vi "CalibrateDistanceCameraSyringe.vi"(5 ".NET Refnum in":refnum<k24>, 6 "error in":errorcluster, 7 "Image Feed":T6, 8 "Template Path":path=path "C:/Users/Aerotech/Documents/BNL_ThermomechanicalStave/1_ModulePlacement", 9 "um/pix resolution":dbl=1.5800403213058958, 10 "Axis speeds (mm/s)":T5={"vX [mm]"=20.0, "vY [mm]"=20.0, "vZ [mm] "=20.0}, 11 "Path to save collected images":path=path "C:/Users/Aerotech/cernbox/BNL/Stave Assembly Records/2017-05-12") -> (0 "X/Y difference (CAMERA - SYRINGE)":dbl[][](array[numeric])=[[-130.04319981335846, 7.799950189407227], [-133.07688928470915, 5.629009425384126]], 3 "XYZ .NET Refnum out":refnum<k24>, 4 "error out":errorcluster={"status"=FALSE, "code"=1073676418, "source"="VISA Close in CalibrateDistanceCameraSyringe.vi"})   [LabVIEW 2016]
uses:
  <vilib>/LabVIEW Interface for Arduino/Type Defs/Arduino Resource.ctl
  <vilib>/LabVIEW Interface for Arduino/Type Defs/Board Type.ctl
  C:/Users/Aerotech/Documents/BNL_ThermomechanicalStave/AerotechLibraries/Bin/Aerotech.A3200.dll
  AerotechLibraries/Bin/Aerotech.A3200.dll
  <vilib>/vision/Measure.llb/Edge Options.ctl
  <vilib>/vision/Measure.llb/Edge Polarity.ctl
  <vilib>/vision/Image Controls.llb/IMAQ Image.ctl
  <vilib>/userdefined/High Color/IMAQdx.ctl
  <vilib>/LabVIEW Interface for Arduino/Type Defs/Pin Mode.ctl
  <vilib>/LabVIEW Interface for Arduino/LabVIEW Interface for Arduino.lvlib
  <vilib>/vision/NI_Vision_Development_Module.lvlib
  <vilib>/vision/driver/NI_Vision_Acquisition_Software.lvlib
panel:
  in  "?":T1(tab)=enum."Results and Error Handling"
  in  "Off stave position":T2={"X [mm]"=250.0, "Y [mm]"=-110.0, "Z [mm] "=26.0}
  in  "Estimate distance x":dbl=132.0
  in  "Estimate distance y":dbl=4.0
  in  "Camera Z":dbl=-24.0
  out "XYZ Stage Control":refnum<k24>
  out "Arduino Resource":T3={"VISA resource"="COM4", "Board Type"=enum."Uno", "Connection Type"=enum."USB / Serial", "Bytes Per Packet (15)"=15}
  in  "Digital I/O Pin":u8=7
  in  "Lowest Z Position":dbl=46.0
  out "Template Image":T6
  out "Camera session out":T7="cam1"
  in  "Camera Name":T7="cam1" caption="IMAQdx Session"
  in  "Testing?":bool
  in  "Circle Finding Options":T10={"Search  Direction"=1, "Edge Options"={"Edge Polarity"=2, "Kernel Size"=3, "Width"=3, "Minimum Edge Strength"=10.0, "Interpolation Type"=enum."Bilinear Fixed", "Data Processing Method"=enum."Median"}, "Show Search Area"=FALSE, "Show Search Lines"=FALSE, "Show Edges Found"=FALSE, "Show Result"=TRUE, "Search Area Color"=65280, "Search Lines Color"=255, "Edge Locations Color"=16776960, "Result Color"=65511, "Overlay Group Name"=""} {"Search  Direction" items=["Outside to Inside", "Inside to Outside"]; "Edge Options"."Edge Polarity" items=["All Edges", "Rising Edges", "Falling Edges"]; "Edge Options"."Minimum Edge Strength" format="%.2f"; "Edge Options"."Width" step=2; "Edge Options"."Kernel Size" step=2}
  in  "Circle ROI Descriptor":T11={"Global Rectangle"=[675, 567, 1751, 1642], "Contours"=[{"ID"=enum."External", "Type"=7, "Coordinates"=[1212, 1104, 85, 537, 0, 0]}]} {"Contours"."Type" items=["No Selection", "Point", "Line", "Rectangle", "Oval", "Polygon", "Freehand Region", "Annulus", "Unused2", "Unused3", "Broken Line", "Freehand Line", "Rotated Rectangle"]}
  in  "Pattern Match Settings":T12={"Algorithm"=2, "Number of Matches Requested"=1, "Minimum Match Score"=100.0, "SubPixel Accuracy"=TRUE, "Rotation Angle Ranges"=[{"Start"=0.0, "End"=360.0}], "Show Search Area"=FALSE, "Show Result"=TRUE} {"Rotation Angle Ranges"."End" format="%.1f"; "Rotation Angle Ranges"."Start" format="%.1f"; "Minimum Match Score" min=0 max=1000 format="%.2f"; "Number of Matches Requested" min=1; "Algorithm" items=["All", "Low Discrepancy Sampling", "Grayscale Value Pyramid", "Gradients Pyramid"]}
  in  "Circle Fit Options":T13={"Process"=enum."Get Best Edge", "Step Size"=3.0, "Max Pixel Radius"=3}
  in  "Fit Circle?":bool
  out "Number of Matches":i32=1
  out "Estimate location":T2={"X [mm]"=118.0, "Y [mm]"=-106.0, "Z [mm] "=-24.0}
  out "pixels x":dbl=1920.0
  out "pixels y":dbl=1374.0
  out "Dot image":T6(plugin-control)
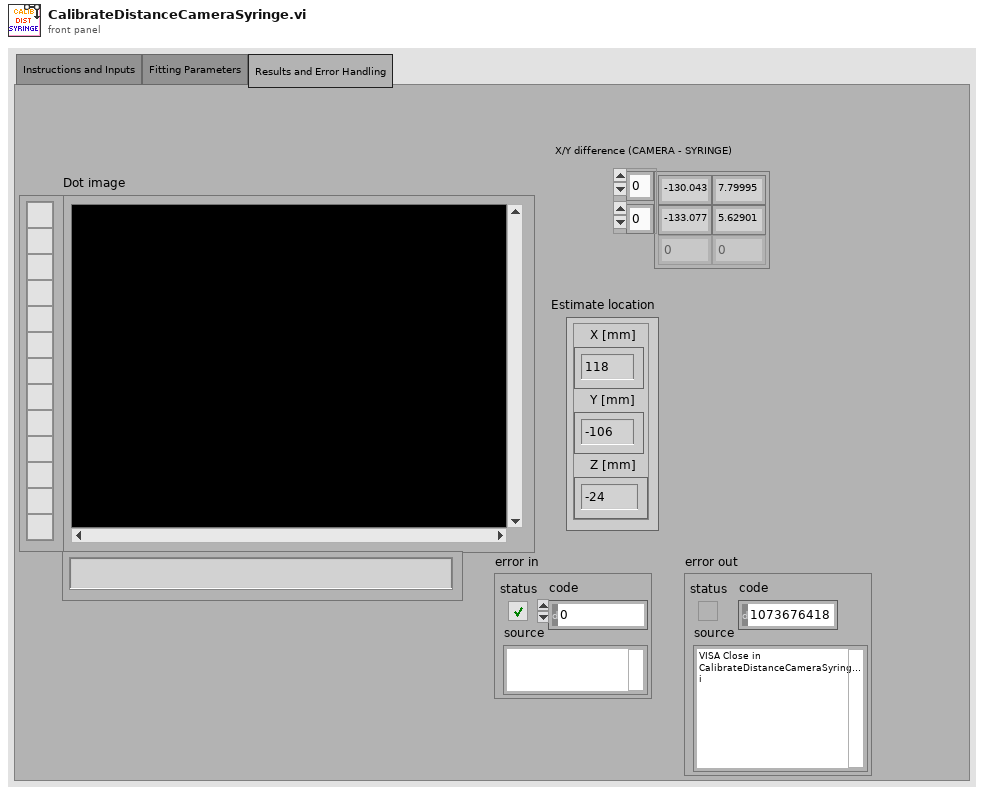
[diagram p1: front panel]
types:
  T1 = enum32{"Instructions and Inputs", "Fitting Parameters", "Results and Error Handling"}
  T2 = cluster{"X [mm]":dbl, "Y [mm]":dbl, "Z [mm] ":dbl}
  T3 = typedef "LabVIEW Interface for Arduino.lvlib/Arduino Resource.ctl" = cluster{"VISA resource":refnum<visa-resource-name>, "Board Type":T4, "Connection Type":enum8{"USB / Serial"}, "Bytes Per Packet (15)":u8}
  T4 = typedef "LabVIEW Interface for Arduino.lvlib/Board Type.ctl" = enum16{"Uno", "Dimuelanove w/Atmega 328", "Mega 2560"}
  T5 = cluster{"vX [mm]":dbl, "vY [mm]":dbl, "vZ [mm] ":dbl}
  T6 = typedef "IMAQ Image.ctl" = refnum<image>
  T7 = typedef "IMAQdx.ctl" = refnum<k21>
  T8 = typedef "Edge Options.ctl" = cluster{"Edge Polarity":T9, "Kernel Size":u32, "Width":u32, "Minimum Edge Strength":sgl, "Interpolation Type":enum32{"Zero Order", "Bilinear", "Quadratic", "Cubic", "Bilinear Fixed"}, "Data Processing Method":enum32{"Average", "Median"}}
  T9 = typedef "Edge Polarity.ctl" = u32
  T10 = cluster{"Search  Direction":u32, "Edge Options":T8, "Show Search Area":bool, "Show Search Lines":bool, "Show Edges Found":bool, "Show Result":bool, "Search Area Color":u32, "Search Lines Color":u32, "Edge Locations Color":u32, "Result Color":u32, "Overlay Group Name":string}
  T11 = cluster{"Global Rectangle":i32[], "Contours":cluster{"ID":enum32{"External", "Internal"}, "Type":u32, "Coordinates":i32[]}[]}
  T12 = cluster{"Algorithm":i32, "Number of Matches Requested":i32, "Minimum Match Score":sgl, "SubPixel Accuracy":bool, "Rotation Angle Ranges":cluster{"Start":sgl, "End":sgl}[], "Show Search Area":bool, "Show Result":bool}
  T13 = cluster{"Process":enum16{"Get First Edge", "Get First + Last Edge", "Get All Edges", "Get Best Edge"}, "Step Size":dbl, "Max Pixel Radius":i32}
  T14 = typedef "LabVIEW Interface for Arduino.lvlib/Pin Mode.ctl" = enum8{"Input", "Output"}
  T15 = typedef "Image Type" = u32
  T16 = cluster{"X [mm]":dbl, "Y [mm]":dbl, "Lowest Z Position":dbl}
  T17 = cluster{"Image Dst Out":T6, "Axis speeds (mm/s)":cluster{"vX [mm]":dbl, "vY [mm]":dbl, "vZ [mm] ":dbl}, ".NET Refnum out":refnum<k24>}
  T18 = cluster{"Captured positions":dbl[][], "XYZ .NET Refnum out":refnum<k24>}
  T19 = cluster{"Position":cluster{"x":sgl, "y":sgl}, "Angle":sgl, "Scale":sgl, "Score":sgl, "Bounding Box":cluster{"x":sgl, "y":sgl}[]}[]
  T20 = cluster{"Position":cluster{"x":sgl, "y":sgl}, "Angle":sgl, "Scale":sgl, "Score":sgl, "Bounding Box":cluster{"x":sgl, "y":sgl}[]}
  T21 = cluster{"Global Rectangle":i32[], cluster{"ID":enum32{"External", "Internal"}, "Type":u32, "Coordinates":i32[]}[]}
  T22 = cluster{"Center (Pixels)":cluster{"X":sgl, "Y":sgl}, "Radius (Pixels)":dbl, "Center (Real-World)":cluster{"X":sgl, "Y":sgl}, "Radius (Real-World)":dbl, "Roundness (Real-World)":dbl, "Average Strength":dbl, "Average SNR (dB)":dbl}
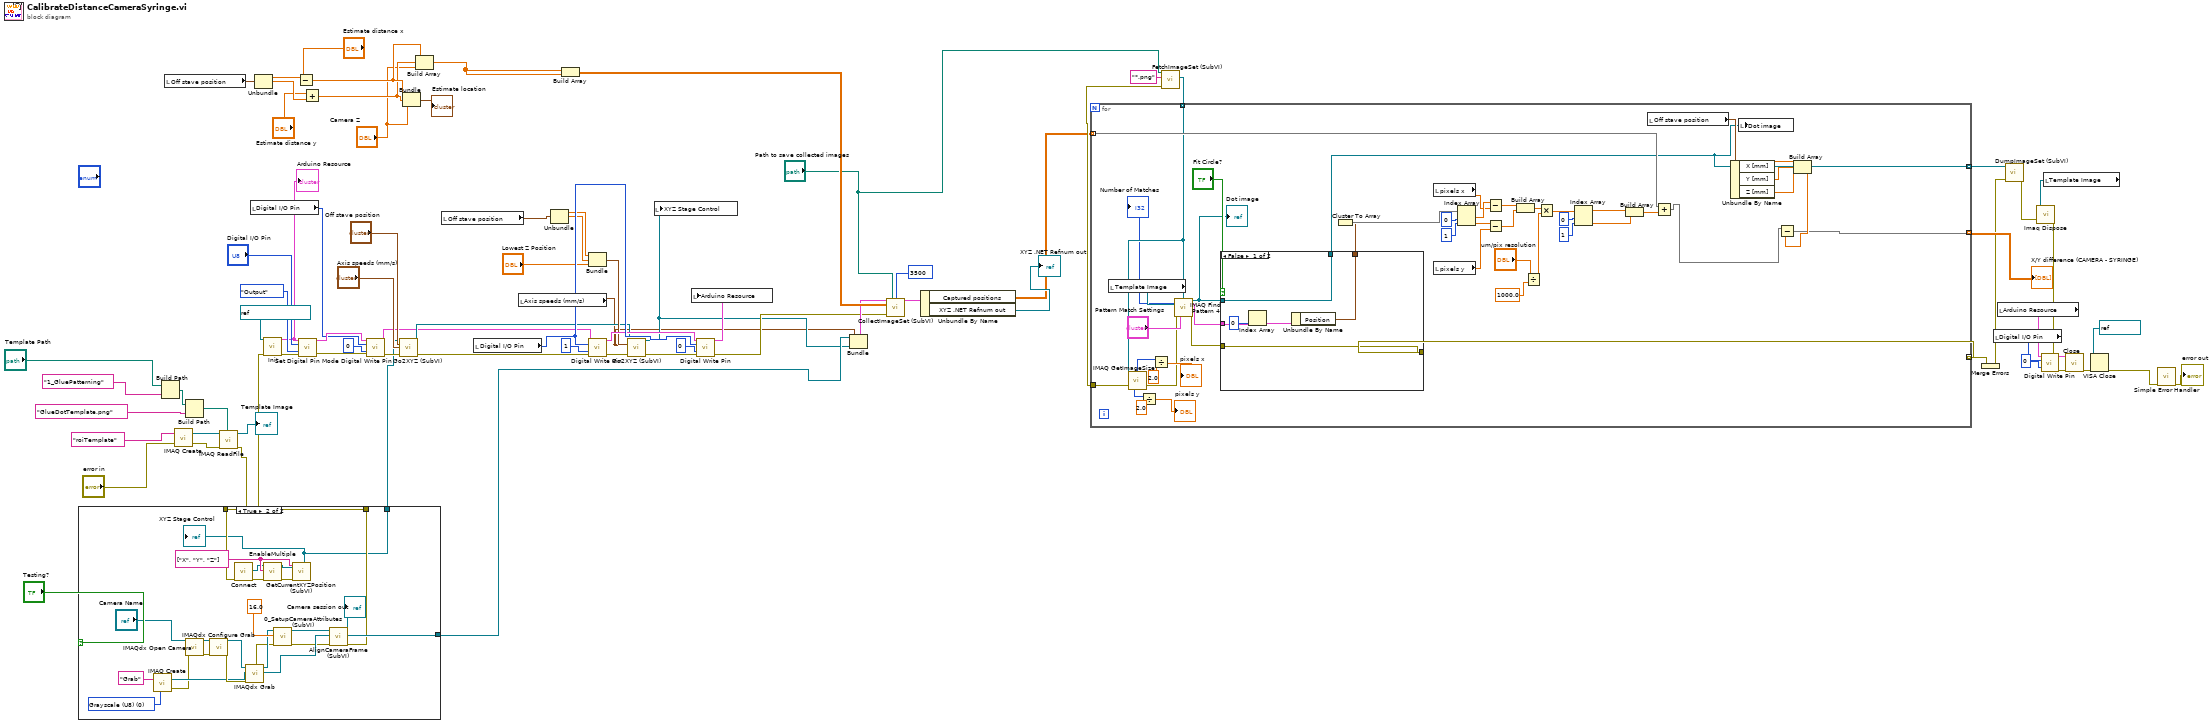
[diagram p0: block diagram]
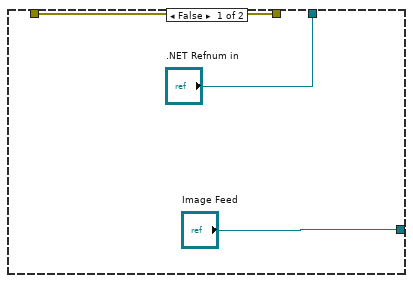
[diagram p2: hidden frame]
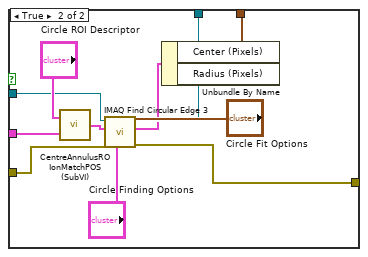
[diagram p3: hidden frame]
diagram:
  n1 = Build Path(base path="Template Path", name or relative path="1_GluePatterning") -> (appended path=w44:path)
  n2 = local read "Off stave position"() -> (w58:T2)
  n3 = call "IMAQ Create"("Image Name"="roiTemplate", "error in (no error)"="error in") -> ("New Image"=w47:T6, "error out"=w48:errorcluster)  [unwired: 3 in]
  n4 = Build Path(base path=w44, name or relative path="GlueDotTemplate.png") -> (appended path=w42:path)
  n5 = call "IMAQ ReadFile"("File Path"=w42, "error in (no error)"=w48, "Image"=w47) -> ("error out"=w22:errorcluster, "Image Out"=→"Template Image":T6)  [unwired: 4 in, 3 out]
  n6 = case shown="True" "Testing?" {
    tunnel: ["Image Feed" w97] -> w31
    tunnel: w22 -> [w84 w89]
    tunnel: [w84 w88] -> w4
    tunnel: [".NET Refnum in" w85] -> w3
    frame False {
    }
    frame True {
      w87 = T15 0 items=["Grayscale (U8)", "Grayscale (I16)", "Grayscale (SGL)", "Complex (CSG)", "RGB (U32)", "HSL (U32)", "RGB (U64)", "Grayscale (U16)"] ("Image Type")
      w93 = string[] ["X", "Y", "Z"] ("Axes Names")
      n7 = call "IMAQ Create"("Image Name"="Grab", "Image Type"=w87) -> ("New Image"=w96:T6, "error out"=w94:errorcluster)  [unwired: 3 in]
      n8 = call <vilib>:"IMAQdx Open Camera.vi"("error in"=w94, "Session In"="Camera Name") -> ("error out"=w107:errorcluster, "Session Out"=w108:T7)  [unwired: 1 in, 7 out]
      n9 = call <vilib>:"IMAQdx Configure Grab.vi"("error in"=w107, "Session In"=w108) -> ("error out"=w100:errorcluster, "Session Out"=w105:T7)  [unwired: 8 out]
      n10 = call "Connect.vi"("error in (no error)"=w89) -> ("error out"=w91:errorcluster, "controller"=w92:refnum<k24>)  [unwired: 9 in]
      n11 = call <vilib>:"IMAQdx Grab.vi"("error in"=w100, "Image In"=w96, "Session In"=w105) -> ("error out"=w99:errorcluster, "Image Out"=w102:T6, "Session Out"=w104:T7)  [unwired: 1 in, 5 out]
      n12 = call "EnableMultiple.vi"("error in (no error)"=w91, "axis names"=w93, "controller in"=w92) -> ("error out"=w90:errorcluster, "controller out"=w86:refnum<k24>)  [unwired: 7 in]
      n13 = call "0_SetupCameraAttributes (SubVI).vi"("error in (no error)"=w99, "Gain"=16.0, "Camera session in"=w104) -> ("error out"=w98:errorcluster, "Camera session out"=w103:T7)  [unwired: 7 in]
      n14 = call "GetCurrentXYZPosition (SubVI).vi"(".NET Refnum in - Device"=w86, "error in (no error)"=w90, "Axes Names"=w93) -> (".NET Refnum out  - Device"=w85:refnum<k24>)  [unwired: 3 in, 5 out]
      "XYZ Stage Control" <- w85
      n15 = call "AlignCameraFrame (SubVI).vi"("error in (no error)"=w98, "Image Src"=w102, "Camera session in"=w103) -> ("error out"=w88:errorcluster, "Image Dst Out"=w97:T6, "Camera session out"=→"Camera session out":T7)  [unwired: 6 in]
    }
  }
  n16 = local read "Digital I/O Pin"() -> (w74:u8)
  n17 = Unbundle(w58) -> ("X [mm]"=w56:dbl, "Y [mm]"=w55:dbl)  [unwired: 1 out]
  n18 = call <vilib>:"Init.vi"("VISA resource"=refnum<visa-resource-name> "COM4", "error in"=w4) -> ("Arduino Resource"=w73:T3, "error out"=w75:errorcluster)  [unwired: 16 in]
  "Arduino Resource" <- w73
  n19 = Subtract(x=w56, y="Estimate distance x") -> (x-y=w51:dbl)
  n20 = call <vilib>:"Set Digital Pin Mode.vi"("Arduino Resource"=w73, "Digital I/O Pin"="Digital I/O Pin", "Pin Mode (Input)"=Pin_Mode."Output", "error in"=w75) -> ("Arduino Resource"=w78:T3, "error out"=w79:errorcluster)  [unwired: 10 in]
  n21 = Add(x="Estimate distance y", y=w55) -> (x+y=w50:dbl)
  n22 = call <vilib>:"Digital Write Pin.vi"("Arduino Resource"=w78, "Digital I/O Pin (0)"=w74, "Value (0)"=u8 0, "error in"=w79) -> ("Arduino Resource"=w38:T3, "error out"=w70:errorcluster)  [unwired: 10 in]
  n23 = call "Go2XYZ (SubVI).vi"(".NET Refnum in"=w3, "Go to Coordinates"="Off stave position", "Axis Speeds"="Axis speeds (mm/s)", "error in (no error)"=w70) -> (".NET Refnum out"=w39:refnum<k24>, "error out"=w66:errorcluster)  [unwired: 7 in, 3 out]
  n24 = Bundle(w51, w50, "Camera Z"="Camera Z") -> (→"Estimate location":cluster{dbl, dbl, "Camera Z":dbl})  [unwired: 1 in]
  n25 = Build Array(w51, w50, "Camera Z") -> (w34:dbl[])
  n26 = local read "Off stave position"() -> (w63:T2)
  n27 = local read "Digital I/O Pin"() -> (w68:u8)
  n28 = local read "Axis speeds (mm/s)"() -> (w19:T5)
  n29 = Unbundle(w63) -> ("X [mm]"=w62:dbl, "Y [mm]"=w61:dbl)  [unwired: 1 out]
  n30 = Build Array(w34, w34) -> (w33:dbl[][])
  n31 = Bundle("X [mm]"=w62, "Y [mm]"=w61, "Lowest Z Position"="Lowest Z Position") -> (w64:T16)  [unwired: 1 in]
  n32 = call <vilib>:"Digital Write Pin.vi"("Arduino Resource"=w38, "Digital I/O Pin (0)"=w68, "Value (0)"=u8 1, "error in"=w66) -> ("Arduino Resource"=w67:T3, "error out"=w59:errorcluster)  [unwired: 10 in]
  n33 = call "Go2XYZ (SubVI).vi"(".NET Refnum in"=w39, "Go to Coordinates"=w64, "Axis Speeds"=w19, "error in (no error)"=w59) -> (".NET Refnum out"=w20:refnum<k24>, "error out"=w69:errorcluster)  [unwired: 7 in, 3 out]
  n34 = local write "XYZ Stage Control"(w20) -> ()
  n35 = call <vilib>:"Digital Write Pin.vi"("Arduino Resource"=w67, "Digital I/O Pin (0)"=w68, "Value (0)"=u8 0, "error in"=w69) -> ("Arduino Resource"=w37:T3, "error out"=w21:errorcluster)  [unwired: 10 in]
  n36 = local write "Arduino Resource"(w37) -> ()
  n37 = Bundle("Image Dst Out"=w31, "Axis speeds (mm/s)"=w19, ".NET Refnum out"=w20) -> (w32:T17)  [unwired: 1 in]
  n38 = call "CollectImageSet (SubVI).vi"("Inputs"=w32, "Path to save collected images"="Path to save collected images", "milliseconds to wait"=u32 3500, "Set of coordinates to process"=w33, "error in"=w21) -> ("Outputs"=w29:T18)  [unwired: 8 in, 2 out]
  n39 = Unbundle By Name(w29) -> ("Captured positions"=w24:dbl[][], "XYZ .NET Refnum out"=→"XYZ .NET Refnum out":refnum<k24>)
  n40 = call "FetchImageSet (SubVI).vi"("Naming Convention"="*.png", "Images Directory"="Path to save collected images") -> ("error out"=w25:errorcluster, "Image Array"=w26:T6[])  [unwired: 7 in, 1 out]
  n41 = for {
    tunnel: w25 -> [w122]
    tunnel: w26 -> [w118] mode=indexing
    tunnel: w24 -> [w120] mode=indexing
    tunnel: [w111] -> w23 mode=indexing
    tunnel: [w116] -> w9 mode=indexing
    tunnel: [w110] -> w11 mode=indexing
    n42 = local read "Template Image"() -> (w125:T6)
    n43 = call "IMAQ GetImageSize"("Image"=w118, "error in (no error)"=w122) -> ("Y Resolution"=w134:i32, "X Resolution"=w131:i32, "error out"=w123:errorcluster)  [unwired: 2 in]
    n44 = Divide(x=w134, y=2.0) -> (x/y=→"pixels y":dbl)
    n45 = Divide(x=w131, y=2.0) -> (x/y=→"pixels x":dbl)
    n46 = call "IMAQ Find Pattern 4"("Image"=w118, "Template"=w125, "error in"=w123, "Settings"="Pattern Match Settings") -> ("Number of Matches"=→"Number of Matches":i32, "Image Out"=w113:T6, "Matches (pixel)"=w137:T19, "error out"=w136:errorcluster)  [unwired: 5 in, 3 out]
    "Dot image" <- w113
    n47 = case shown="False" "Fit Circle?" {
      tunnel: w113 -> [w161 w168]
      tunnel: w137 -> [w159 w167]
      tunnel: w136 -> [w160 w166]
      tunnel: [w161 w165] -> w110
      tunnel: [w160 w164] -> w116
      tunnel: [w156 w162] -> w114
      frame False {
        n48 = Index Array(array=w159, index=0) -> (element=w157:T20)
        n49 = Unbundle By Name(w157) -> ("Position"=w156:cluster{"x":sgl, "y":sgl})
      }
      frame True {
        n50 = call "CentreAnnulusROIonMatchPOS (SubVI).vi"("Matches (pixel)"=w167, "Annulus ROI Descriptor"="Circle ROI Descriptor") -> ("Annulus ROI Descriptor centred on match position"=w169:T21)
        n51 = call "IMAQ Find Circular Edge 3"("Circle Fit Options"="Circle Fit Options", "Options"="Circle Finding Options", "error in (no error)"=w166, "ROI Descriptor"=w169, "Image"=w168) -> ("error out"=w164:errorcluster, "Fitted Circle"=w163:T22, "Image Out"=w165:T6)  [unwired: 2 in, 2 out]
        n52 = Unbundle By Name(w163) -> ("Center (Pixels)"=w162:cluster{"X":sgl, "Y":sgl})  [unwired: 1 out]
      }
    }
    n53 = Cluster To Array(cluster=w114) -> (array=w146:sgl[])
    n54 = local read "pixels x"() -> (w141:dbl)
    n55 = local read "pixels y"() -> (w142:dbl)
    n56 = Index Array(array=w146, index #1=0 ("index"), index #2=1 ("index")) -> (element #1=w147:sgl, element #2=w143:sgl)
    n57 = Subtract(x=w147, y=w141) -> (x-y=w149:dbl)
    n58 = Subtract(x=w143, y=w142) -> (x-y=w148:dbl)
    n59 = Build Array(w149, w148) -> (w140:dbl[])
    n60 = Divide(x="um/pix resolution", y=1000.0) -> (x/y=w150:dbl)
    n61 = Multiply(x=w140, y=w150) -> (x*y=w155:dbl[])
    n62 = Index Array(array=w155, index #1=0, index #2=1) -> (element #1=w139:dbl, element #2=w138:dbl)
    n63 = Build Array(w139, w138) -> (w121:dbl[])
    n64 = local read "Off stave position"() -> (w129:T2)
    n65 = Add(x=w120, y=w121) -> (x+y=w126:dbl[])
    n66 = Unbundle By Name(w129) -> ("X [mm]"=w128:dbl, "Y [mm]"=w127:dbl, "Z [mm]"=w117:dbl)
    n67 = local write "Dot image"(w110) -> ()
    n68 = Build Array(w128, w127, w117) -> (w119:dbl[])
    n69 = Subtract(x=w126, y=w119) -> (x-y=w111:dbl[])
  }
  "X/Y difference (CAMERA - SYRINGE)" <- w23
  n70 = Merge Errors(w9) -> (w8:errorcluster)
  n71 = local read "Digital I/O Pin"() -> (w14:u8)
  n72 = local read "Arduino Resource"() -> (w13:T3)
  n73 = call "DumpImageSet (SubVI).vi"("error in (no error)"=w8, "Calibrated Image Array"=w11) -> ("error out"=w7:errorcluster)  [unwired: 6 in]
  n74 = local read "Template Image"() -> (w10:T6)
  n75 = call "Imaq Dispose"("Image"=w10, "error in (no error)"=w7) -> ("error out"=w6:errorcluster)  [unwired: 4 in]
  n76 = call <vilib>:"Digital Write Pin.vi"("Arduino Resource"=w13, "Digital I/O Pin (0)"=w14, "Value (0)"=u8 0, "error in"=w6) -> ("Arduino Resource"=w17:T3, "error out"=w16:errorcluster)  [unwired: 10 in]
  n77 = call <vilib>:"Close.vi"("Arduino Resource"=w17, "error in"=w16) -> ("error out"=w15:errorcluster)  [unwired: 13 in]
  n78 = VISA Close(VISA resource name=refnum<visa-resource-name> "COM4", error in (no error)=w15) -> (error out=w2:errorcluster)
  n79 = call <vilib>:"Simple Error Handler.vi"("error in (no error)"=w2) -> ("error out"=→"error out":errorcluster)  [unwired: 4 in, 4 out]
